vi "Async Engine.vi"(10 "Parameters":variant, 11 "Process":refnum<class "Process.lvclass">) -> ()   [LabVIEW 2015, in "Fuel Injection Addon Engine.lvlib"]
uses:
  Fuel Injection Addon Engine.lvlib
  <vilib>/NI/NIVS Inline Async API/_VS Inline Async API/Process/Process.lvclass
  Types/Async Parameters.ctl
  Shared/Types/Injector info.ctl
  Shared/Types/Shot.Parameters.ctl
  Shared/Types/Stage.Parameters.ctl
  Shared/Types/Stage.PullIn.Types.ctl
  Shared/Types/Stage.Transition.Types.ctl
  <vilib>/NI Veristand/Custom Device API/Waveform Data Reference.ctl
  <vilib>/NI VeriStand/Custom Device Waveform API/Single Waveform Write (DBL)/Single Waveform Write (DBL).lvclass
  <vilib>/NI/NIVS Inline Async API/_Data Access Engine/Data Access Engine/Types/Read.DVR.ctl
  <vilib>/NI/NIVS Inline Async API/_Data Access Engine/Access Type Classes/Read/Read.lvclass
  <vilib>/NI/NIVS Inline Async API/_Data Access Engine/Data Access Engine/Types/Write.DVR.ctl
  <vilib>/NI/NIVS Inline Async API/_Data Access Engine/Access Type Classes/Write/Write.lvclass
  Shared/Types/Analysis.Channels.Select.ctl
  <vilib>/NI/NIVS Inline Async API/_VS Inline Async API/Process/Process.lvclass/Process.ctl
  <vilib>/Platform/TimedLoop/XDataNode/timing_clust.ctl
  <vilib>/Platform/TimedLoop/XDataNode/nitl_modes.ctl
  <vilib>/Platform/TimedLoop/XDataNode/wakeup.ctl
  <vilib>/NI/NIVS Inline Async API/_Data Access Engine/Access Type Classes/Write/Write.lvclass/Write.ctl
  <vilib>/NI/NIVS Inline Async API/_Data Access Engine/Data Access Engine/Methods/Write.Data.vi
  <vilib>/NI/NIVS Inline Async API/_VS Inline Async API/Process/Data Member Access/Read Data Access.vi
  <vilib>/NI/NIVS Inline Async API/_VS Inline Async API/Error Handling Process/SubVIs/Error.ConvertArray.vi
  <vilib>/NI/NIVS Inline Async API/_Data Access Engine/Access Type Classes/Write/Write.ProcessData.vi
  <vilib>/NI/NIVS Inline Async API/_Data Access Engine/Data Access Engine/Methods/Write.Lookup.vi
  <vilib>/NI/NIVS Inline Async API/_Data Access Engine/Data Access Engine/Methods/Read.Lookup.vi
  <vilib>/NI Veristand/Custom Device Waveform API/NI VeriStand - Open Waveform Session.vi
  <vilib>/NI Veristand/Custom Device Waveform API/Single Waveform Write (DBL)/NI VeriStand - Open Single Waveform Write Session (DBL).vi
  Shared/Constants.vi
  <vilib>/Platform/TimedLoop/XDataNode/XDataNode.xnode
  <vilib>/NI/NIVS Inline Async API/_Data Access Engine/Data Access Engine/Data Access Engine.lvclass
  <vilib>/NI Veristand/Custom Device Tools/Custom Device Utility Library/Custom Device Utility Library.lvlib
  Shared/Fuel Injection Addon Shared.lvlib
  <vilib>/NI VeriStand/Custom Device API/Custom Device API.lvlib
  <vilib>/Platform/TimedLoop/XDataNode/XDNodeRunTimeDep.lvlib
panel:
  in  "Error":errorcluster
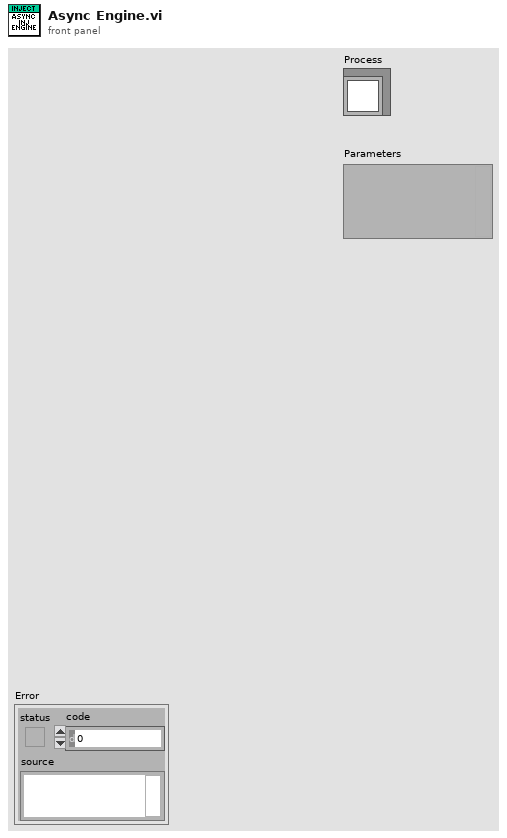
[diagram p1: front panel]
types:
  T1 = typedef "Fuel Injection Addon Engine.lvlib/Async Parameters.ctl" = cluster{"Name":string, "Rate.Hz":u32, "Injectors.Count":u8, "Injector.Timeout":dbl, "Injector.Timer":u32[], "Injector.Info":T2[], "Events.Count":u64[], "Event.Parameters":T3, "DMA.Ref":refnum<k20>, "Waveform.Refs":T7[], "Waveform.Sessions":refnum<class "Single Waveform Write (DBL).lvclass">[], "Waveform.Enable":T8, "FPGA.Status":T9, "Search.Data":T8, "Results.Data":T9, "Results.Values":dbl[], "Results.Selections":T10[]}
  T2 = typedef "Fuel Injection Addon Shared.lvlib/Injector info.ctl" = cluster{"Results Index":i32, "Waveform Index":i32}
  T3 = typedef "Fuel Injection Addon Shared.lvlib/Shot.Parameters.ctl" = cluster{"Shots":u32, "Shot.InitialVoltage":dbl, "Shot.Stages":u32, "Stages":T4[]}
  T4 = typedef "Fuel Injection Addon Shared.lvlib/Stage.Parameters.ctl" = cluster{"Stage.Dwell.Level":dbl, "PullIn.Type":T5, "PullIn.Level":dbl, "Transition.Type":T6, "Transition.Level":dbl}
  T5 = typedef "Fuel Injection Addon Shared.lvlib/Stage.PullIn.Types.ctl" = enum8{"Pull In Transition Dwells", "Pull In Transition Current Drop"}
  T6 = typedef "Fuel Injection Addon Shared.lvlib/Stage.Transition.Types.ctl" = enum8{"Stage Transition Dwell Time", "Stage Transition Voltage Level", "Stage Transition Current Drop"}
  T7 = typedef "Custom Device API.lvlib/Waveform Data Reference.ctl" = i32
  T8 = typedef "Data Access Engine.lvlib/Data Access Engine.lvclass/Read.DVR.ctl" = refnum<data-value>
  T9 = typedef "Data Access Engine.lvlib/Data Access Engine.lvclass/Write.DVR.ctl" = refnum<data-value>
  T10 = typedef "Fuel Injection Addon Shared.lvlib/Analysis.Channels.Select.ctl" = cluster{"Pull In Time":bool, "Pull In Max Current":bool, "Hold In Time":bool, "Hold In Max Current":bool, "Hold In Min Current":bool, "Hold In Avg Current":bool, "Hold In Avg Max Current":bool, "Hold In Avg Min Current":bool, "Hold In Max Voltage":bool, "Hold In Min Voltage":bool, "Hold In Avg Voltage":bool, "Hold In Avg Max Voltage":bool, "Hold In Avg Min Voltage":bool, "Off Time":bool, "Off Stage Max Current":bool, "Off Stage Min Current":bool, "Off Stage Avg Current":bool, "Total Voltage Pulses":bool}
  T11 = typedef "Fuel Injection Addon Engine.lvlib/Injector Event Data Cluster.ctl" = cluster{"Injector.Current":i16, "Injection.Period":dbl, "Shots":T12[], "Shots.Count":i32, "Current.Values":dbl[], "Voltage.Values":dbl[]}
  T12 = typedef "Fuel Injection Addon Engine.lvlib/Shot Information Control.ctl" = cluster{"Transition.Array":i32[], "Stages.Found":u16, "Results":T13[], "Shot.Time":dbl, "FPGA Shot Time (ms)":dbl}
  T13 = typedef "Fuel Injection Addon Engine.lvlib/Stage.Measurements.ctl" = cluster{"Pull-In Time (us)":dbl, "Pull-In Max Current":dbl, "Hold-In Time (us)":dbl, "Hold-In Max Current":dbl, "Hold-In Min Current":dbl, "Hold-In Avg Current":dbl, "Hold-In Avg Max Current":dbl, "Hold-In Avg Min Current":dbl, "Hold-In Max Volt":dbl, "Hold-In Min Volt":dbl, "Hold-In Avg Volt":dbl, "Hold-In Avg Max Volt":dbl, "Hold-In Avg Min Volt":dbl, "Off-Stage Time (us)":dbl, "Off-Stage Max Current":dbl, "Off-Stage Min Current":dbl, "Off-Stage Avg Current":dbl, "Total Voltage Pulses":dbl}
  T14 = typedef "XDNodeRunTimeDep.lvlib/timing_clust.ctl" = cluster{"Expected End [f-1]":u64, "Actual End [f-1]":u64, "Finished Late? [f-1]":bool, "Expected End [i-1]":u64, "Actual End [i-1]":u64, "Finished Late? [i-1]":bool, "Expected Start [i]":u64, "Actual Start [i]":u64, "Expected Start [f]":u64, "Actual Start [f]":u64, "Source Name":string, "Structure Name":string, "Period":i64, "Deadline":i64, "Offset":i64, "Start":i64, "Priority":i32, "Timeout":i32, "Mode":T15, "Wakeup Reason":T16, "Error":errorcluster, "Source Type":string, "Secondary Source Type":string, "Global End Time":u64, "Global Start Time":u64, "Frame Duration":u64, "Iteration Duration":u64, "Assigned CPU":i32, "I/O Scan Engine Mode":u32}
  T15 = typedef "XDNodeRunTimeDep.lvlib/nitl_modes.ctl" = enum32{"No Change", "Process missed periods, maintain original phase", "Discard missed periods, maintain original phase", "Process missed periods, ignore original phase", "Discard missed periods, ignore original phase"}
  T16 = typedef "XDNodeRunTimeDep.lvlib/wakeup.ctl" = enum32{"Normal", "Aborted", "Asynchronous wakeup", "Timing source error", "Timed loop error", "Timeout"}
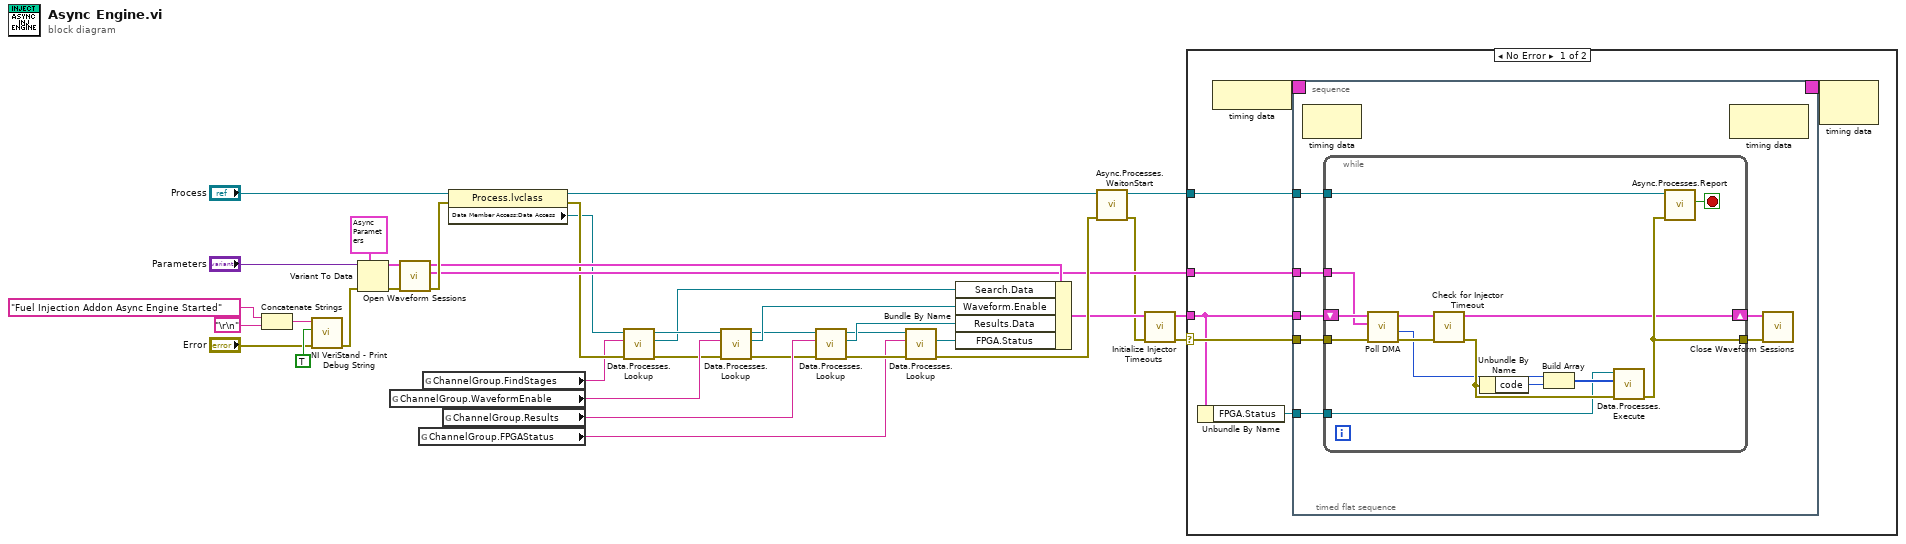
[diagram p0: block diagram]
diagram:
  n1 = Concatenate Strings("Fuel Injection Addon Async Engine Started" ("Message"), "\r\n") -> (w34:string)
  n2 = call <vilib>:"NI VeriStand - Print Debug String.vi"("error in (no error)"="Error", "Add to log file? (T)"=TRUE, "Message"=w34) -> ("error out"=w30:errorcluster)  [unwired: 8 in]
  n3 = Variant To Data(error in=w30, type=T1 {"Name"="", "Rate.Hz"=0, "Injectors.Count"=0, "Injector.Timeout"=0.0, "Injector.Timer"=[], "Injector.Info"=[], "Events.Count"=[], "Event.Parameters"={"Shots"=0, "Shot.InitialVoltage"=0.0, "Shot.Stages"=0, "Stages"=[{"Stage.Dwell.Level"=0.0, "PullIn.Type"=enum."Pull In Transition Dwells", "PullIn.Level"=0.0, "Transition.Type"=enum."Stage Transition Voltage Level", "Transition.Level"=0.0}]}, "DMA.Ref"=refnum, "Waveform.Refs"=[], "Waveform.Sessions"=[], "Waveform.Enable"=refnum, "FPGA.Status"=refnum, "Search.Data"=refnum, "Results.Data"=refnum, "Results.Values"=[], "Results.Selections"=[]} ("Parameters"), Variant="Parameters") -> (data=w18:T1, error out=w19:errorcluster)
  n4 = global read "Constants.vi" "ChannelGroup.WaveformEnable"() -> (w25:string)
  n5 = call "Open Waveform Sessions.vi"("error in"=w19, "Parameters"=w18) -> ("error out"=w27:errorcluster, "Injection.Results"=w11:T11, "Parameters"=w26:T1)  [unwired: 7 in]
  n6 = global read "Constants.vi" "ChannelGroup.FPGAStatus"() -> (w13:string)
  n7 = global read "Constants.vi" "ChannelGroup.FindStages"() -> (w2:string)
  n8 = global read "Constants.vi" "ChannelGroup.Results"() -> (w23:string)
  n9 = property class="Process.lvclass"(reference="Process", error in=w27) -> (reference out=w28:refnum<class "Process.lvclass">, error out=w6:errorcluster, "Data Member Access:Data Access"=w4:refnum<class "Data Access Engine.lvclass">)
  n10 = call-poly <vilib>:"Data.Processes.Lookup.vi"("error in (no error)"=w6, "Name"=w2, "Data Access API in"=w4) -> ("error out"=w5:errorcluster, "Ref"=w1:T8, "Data Access API out"=w3:refnum<class "Data Access Engine.lvclass">)  [unwired: 5 in, 1 out]
  n11 = call-poly <vilib>:"Data.Processes.Lookup.vi"("error in (no error)"=w5, "Name"=w25, "Data Access API in"=w3) -> ("error out"=w21:errorcluster, "Ref"=w24:T8, "Data Access API out"=w22:refnum<class "Data Access Engine.lvclass">)  [unwired: 5 in, 1 out]
  n12 = call-poly <vilib>:"Data.Processes.Lookup.vi"("error in (no error)"=w21, "Name"=w23, "Data Access API in"=w22) -> ("error out"=w15:errorcluster, "Ref"=w20:T9, "Data Access API out"=w16:refnum<class "Data Access Engine.lvclass">)  [unwired: 5 in, 1 out]
  n13 = call-poly <vilib>:"Data.Processes.Lookup.vi"("error in (no error)"=w15, "Name"=w13, "Data Access API in"=w16) -> ("error out"=w14:errorcluster, "Ref"=w12:T9)  [unwired: 5 in, 2 out]
  n14 = Bundle By Name(cluster=w26, "Search.Data"=w1, "Waveform.Enable"=w24, "Results.Data"=w20, "FPGA.Status"=w12) -> (w9:T1)
  n15 = call <vilib>:"Async.Processes.WaitonStart.vi"("error in (no error)"=w14, "Process"=w28) -> ("error out"=w8:errorcluster, "Process out"=w17:refnum<class "Process.lvclass">)  [unwired: 7 in, 1 out]
  n16 = call "Initialize Injector Timeouts.vi"("error in (no error)"=w8, "Parameters"=w9) -> ("error out"=w7:errorcluster, "Parameters"=w10:T1)  [unwired: 8 in]
  n17 = case shown="No Error" w7 {
    selector: w7 -> [w40 _]
    tunnel: w10 -> [w39 _]
    tunnel: w17 -> [w44 _]
    tunnel: w11 -> [w41 _]
    frame No Error {
      n18 = Unbundle By Name(w39) -> ("FPGA.Status"=w38:T9)
      n19 = node-c288() -> (w43:T14)
      n20 = timed-sequence {
        timing: w43 -> [_]
        timing-out: [_] -> w42
        tunnel: w39 -> [w49]
        tunnel: w40 -> [w48]
        tunnel: w44 -> [w47]
        tunnel: w41 -> [w46]
        tunnel: w38 -> [w45]
        n21 = timed-flat-sequence {
          tunnel: w49 -> [w56]
          tunnel: w48 -> [w53]
          tunnel: w47 -> [w52]
          tunnel: w46 -> [w51]
          tunnel: w45 -> [w50]
          n22 = node-c288() -> ()  [unwired: 1 in, 1 out]
          n23 = while {
            tunnel: w53 -> [w70]
            shift-right: [w63] -> w54
            shift-left: w56 -> [w61]
            tunnel: [w65] -> w55
            tunnel: w52 -> [w69]
            tunnel: w51 -> [w57]
            tunnel: w50 -> [w58]
            stop <- w68 stop-if-true
            n24 = call "Poll DMA.vi"("error in"=w70, "Injection.Results"=w57, "Parameters"=w61) -> ("error out"=w62:errorcluster, "Elements Remaining"=w60:u32, "Parameters"=w59:T1)  [unwired: 6 in]
            n25 = call "Check for Injector Timeout.vi"("error in (no error)"=w62, "Parameters"=w59) -> ("error out"=w64:errorcluster, "Parameters"=w63:T1)  [unwired: 8 in]
            n26 = Unbundle By Name(w64) -> ("code"=w66:i32)
            n27 = Build Array(w60, w66) -> (w67:u32[])
            n28 = call-poly <vilib>:"Data.Processes.Execute.vi"("error in (no error)"=w64, "Values"=w67, "Ref"=w58) -> ("error out"=w65:errorcluster)  [unwired: 8 in]
            n29 = call <vilib>:"Async.Processes.Report.vi"("Error"=w65, "Process in"=w69) -> ("Stop"=w68:bool)  [unwired: 8 in, 1 out]
          }
          n30 = node-c288() -> ()  [unwired: 1 in, 1 out]
          n31 = call "Close Waveform Sessions.vi"("error in"=w55, "Async Parameters"=w54) -> ()  [unwired: 9 in, 1 out]
        }
      }
      n32 = node-c288(w42) -> ()  [unwired: 1 out]
    }
    frame Error {
    }
  }
